vi "test_libssh2_channel_wait_eof.vi"() -> ()   [LabVIEW 2013, in "libssh2_integration_tests.lvlib"]
uses:
  libssh2_integration_tests.lvlib
  <vilib>/addons/_JKI Toolkits/Caraya/classes/Test/Test.lvclass
  libssh2/libssh2.lvlib
  <vilib>/addons/_JKI Toolkits/Caraya/classes/Assert/Assert.lvclass
panel:
  out "error out":errorcluster
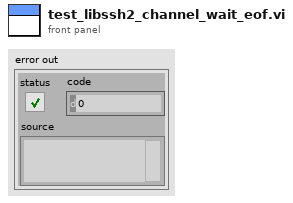
[diagram p1: front panel]
types:
  T1 = typedef "libssh2.lvlib/Session Refnum.ctl" = refnum<k1>
  T2 = typedef "libssh2.lvlib/Channel Refnum.ctl" = refnum<k1>
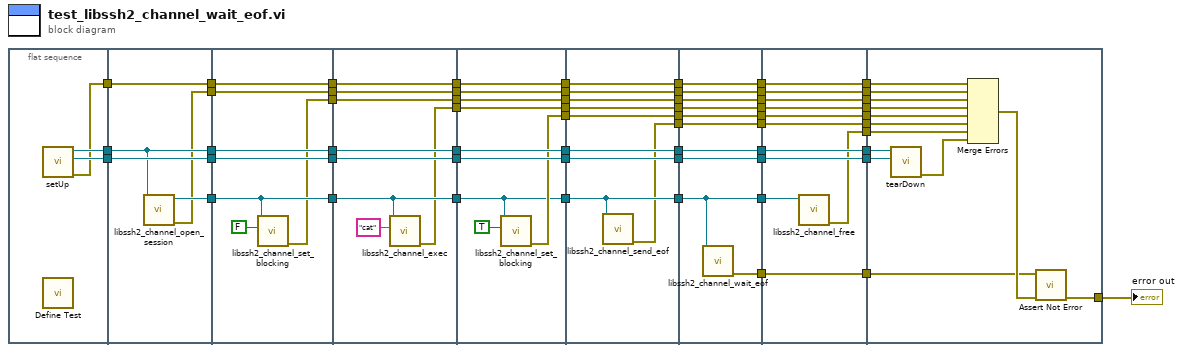
[diagram p0: block diagram]
diagram:
  n1 = flat-sequence {
    tunnel: [w62] -> w59
    tunnel: [w61] -> w58
    tunnel: [w60] -> w57
    tunnel: w59 -> [w66]
    tunnel: w58 -> [w67]
    tunnel: [w66] -> w32
    tunnel: [w67] -> w30
    tunnel: [w65] -> w24
    tunnel: w57 -> [w64]
    tunnel: [w64] -> w28
    tunnel: [w63] -> w26
    tunnel: w32 -> [w74]
    tunnel: [w74] -> w31
    tunnel: w30 -> [w73]
    tunnel: [w73] -> w29
    tunnel: w28 -> [w72]
    tunnel: [w72] -> w27
    tunnel: w26 -> [w71]
    tunnel: [w71] -> w25
    tunnel: w24 -> [w70]
    tunnel: [w70] -> w23
    tunnel: [w68] -> w22
    tunnel: w31 -> [w82]
    tunnel: [w82] -> w18
    tunnel: w29 -> [w81]
    tunnel: [w81] -> w16
    tunnel: w27 -> [w80]
    tunnel: [w80] -> w14
    tunnel: w25 -> [w79]
    tunnel: [w79] -> w12
    tunnel: w23 -> [w78]
    tunnel: [w78] -> w10
    tunnel: [w76] -> w8
    tunnel: w22 -> [w75]
    tunnel: [w75] -> w6
    tunnel: w18 -> [w91]
    tunnel: [w91] -> w17
    tunnel: w16 -> [w90]
    tunnel: [w90] -> w15
    tunnel: w14 -> [w89]
    tunnel: [w89] -> w13
    tunnel: w12 -> [w88]
    tunnel: [w88] -> w11
    tunnel: w10 -> [w83]
    tunnel: [w83] -> w9
    tunnel: w8 -> [w87]
    tunnel: [w87] -> w7
    tunnel: w6 -> [w86]
    tunnel: [w86] -> w5
    tunnel: [w84] -> w4
    tunnel: w17 -> [w100]
    tunnel: [w100] -> w49
    tunnel: w15 -> [w99]
    tunnel: [w99] -> w47
    tunnel: w13 -> [w98]
    tunnel: [w98] -> w45
    tunnel: w11 -> [w97]
    tunnel: [w97] -> w43
    tunnel: w9 -> [w96]
    tunnel: [w96] -> w41
    tunnel: [w95] -> w38
    tunnel: w7 -> [w94]
    tunnel: [w94] -> w35
    tunnel: w5 -> [w93]
    tunnel: [w93] -> w21
    tunnel: w4 -> [w92]
    tunnel: [w92] -> w3
    tunnel: w49 -> [w110]
    tunnel: [w110] -> w48
    tunnel: w47 -> [w109]
    tunnel: [w109] -> w46
    tunnel: w45 -> [w108]
    tunnel: [w108] -> w44
    tunnel: w43 -> [w107]
    tunnel: [w107] -> w42
    tunnel: w41 -> [w105]
    tunnel: [w105] -> w40
    tunnel: [w104] -> w39
    tunnel: w38 -> [w106]
    tunnel: [w106] -> w37
    tunnel: w35 -> [w103]
    tunnel: [w103] -> w34
    tunnel: w21 -> [w102]
    tunnel: [w102] -> w20
    tunnel: w3 -> [w101]
    tunnel: [w101] -> w2
    tunnel: w48 -> [w121]
    tunnel: w46 -> [w120]
    tunnel: [w121] -> w56
    tunnel: [w120] -> w55
    tunnel: [w119] -> w54
    tunnel: w44 -> [w118]
    tunnel: [w118] -> w53
    tunnel: w42 -> [w117]
    tunnel: [w117] -> w52
    tunnel: w40 -> [w116]
    tunnel: w39 -> [w115]
    tunnel: [w115] -> w50
    tunnel: w37 -> [w114]
    tunnel: [w114] -> w36
    tunnel: w34 -> [w113]
    tunnel: [w113] -> w33
    tunnel: w20 -> [w112]
    tunnel: [w112] -> w19
    tunnel: w2 -> [w111]
    tunnel: [w111] -> w1
    tunnel: w56 -> [w134]
    tunnel: w55 -> [w133]
    tunnel: [w132] -> w51
    tunnel: w54 -> [w130]
    tunnel: w53 -> [w129]
    tunnel: w52 -> [w127]
    tunnel: w50 -> [w126]
    tunnel: w36 -> [w125]
    tunnel: w33 -> [w124]
    tunnel: w19 -> [w123]
    tunnel: w1 -> [w122]
    frame #0 {
      n2 = call "setUp.vi"() -> ("error out"=w60:errorcluster, "connection ID"=w61:refnum<k5>, "session"=w62:T1)  [unwired: 9 in]
      n3 = call <vilib>:"Define Test.vi"() -> ()  [unwired: 10 in, 2 out]
    }
    frame #1 {
      n4 = call "libssh2_channel_open_session.vi"("session"=w66) -> ("error out"=w63:errorcluster, "channel"=w65:T2)  [unwired: 9 in]
    }
    frame #2 {
      n5 = call "libssh2_channel_set_blocking.vi"("blocking"=FALSE, "channel"=w70) -> ("error out"=w68:errorcluster)  [unwired: 9 in]
    }
    frame #3 {
      n6 = call "libssh2_channel_exec.vi"("command"="cat", "channel"=w78) -> ("error out"=w76:errorcluster)  [unwired: 9 in]
    }
    frame #4 {
      n7 = call "libssh2_channel_set_blocking.vi"("blocking"=TRUE, "channel"=w83) -> ("error out"=w84:errorcluster)  [unwired: 9 in]
    }
    frame #5 {
      n8 = call "libssh2_channel_send_eof.vi"("channel"=w96) -> ("error out"=w95:errorcluster)  [unwired: 10 in]
    }
    frame #6 {
      n9 = call "libssh2_channel_wait_eof.vi"("channel"=w105) -> ("error out"=w104:errorcluster)  [unwired: 10 in]
    }
    frame #7 {
      n10 = call "libssh2_channel_free.vi"("channel"=w116) -> ("error out"=w119:errorcluster)  [unwired: 10 in]
    }
    frame #8 {
      n11 = call "tearDown.vi"("connection ID"=w133, "session"=w134) -> ("error out"=w131:errorcluster)  [unwired: 9 in]
      n12 = Merge Errors(w129, w127, w123, w124, w122, w125, w130, w131) -> (w128:errorcluster)
      n13 = call <vilib>:"Assert Not Error.vi"("error in (no error)"=w128, "Not Error?"=w126) -> ("error out"=w132:errorcluster)  [unwired: 8 in, 1 out]
    }
  }
  "error out" <- w51
